vi "String Tuning.vi"(8 "Upper Limit":dbl, 9 "Lower Limit":dbl, 10 "Frequency":dynamicdata(waveform), 11 "Cluster in":T1) -> (1 "Tuned":bool, 3 "Cluster out":T1)   [LabVIEW 2020]
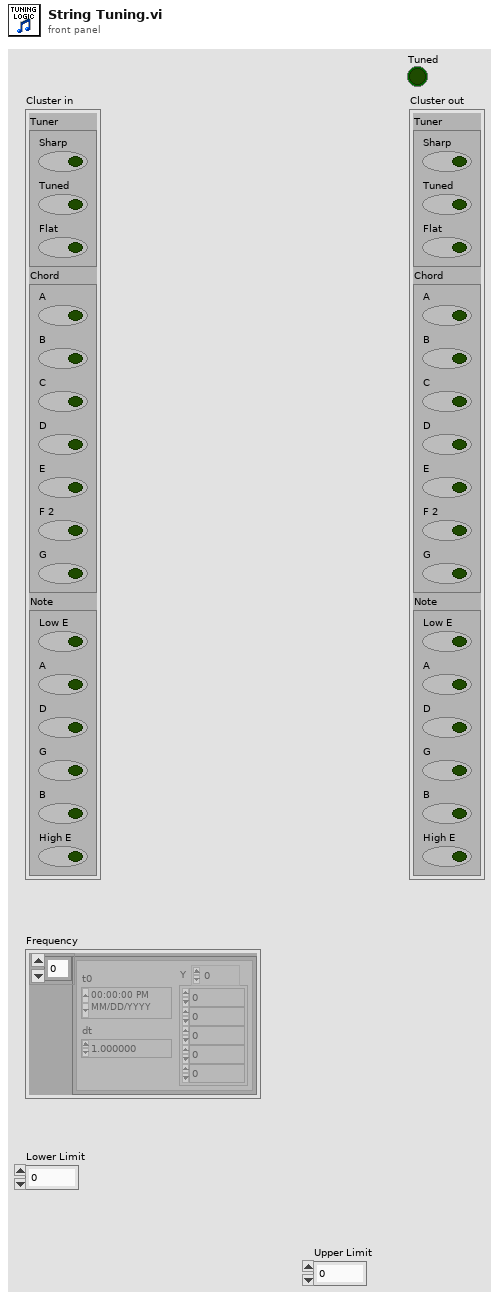
[diagram p1: front panel]
types:
  T1 = cluster{"Tuner":cluster{"Sharp":bool, "Tuned":bool, "Flat":bool}, "Chord":cluster{"A":bool, "B":bool, "C":bool, "D":bool, "E":bool, "F 2":bool, "G":bool}, "Note":cluster{"Low E":bool, "A":bool, "D":bool, "G":bool, "B":bool, "High E":bool}}
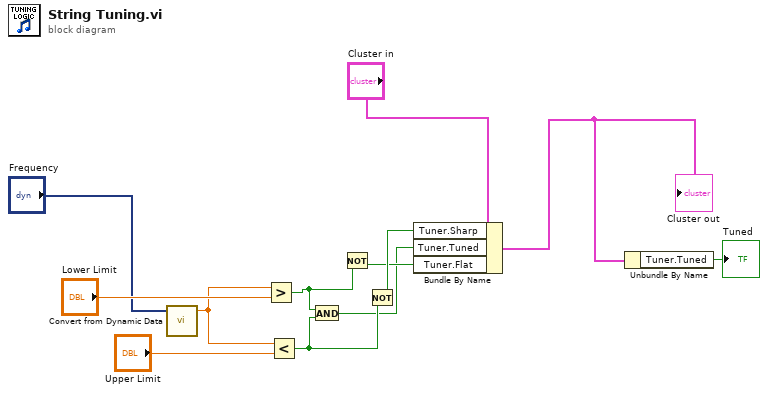
[diagram p0: block diagram]
diagram:
  n1 = call "Convert from Dynamic Data"("Dynamic Data Type"="Frequency") -> ("Scalar"=w4:dbl)  [unwired: 3 in]
  n2 = Greater?(x=w4, y="Lower Limit") -> (0:w9:bool)
  n3 = Less?(x=w4, y="Upper Limit") -> (x < y?=w11:bool)
  n4 = And(x=w9, y=w11) -> (x .and. y?=w8:bool)
  n5 = Not(x=w9) -> (.not. x?=w10:bool)
  n6 = Not(x=w11) -> (.not. x?=w12:bool)
  n7 = Bundle By Name(cluster="Cluster in", "Tuner.Sharp"=w12, "Tuner.Tuned"=w8, "Tuner.Flat"=w10) -> (w2:T1)
  "Cluster out" <- w2
  n8 = Unbundle By Name(w2) -> ("Tuner.Tuned"=→"Tuned":bool)
